vi "Get All DMA Data.vi"(10 "size":u32, 11 "arr":i32) -> (2 "function return":u32, 3 "arr out":i32)   [LabVIEW 2018, in "Copy of Andor SDK.lvlib"]
doc: "EXPNETTYPE unsigned int WINAPI GetAllDMAData(at_32 * arr, unsigned long size);"
uses:
  Copy of Andor SDK.lvlib
  <userlib>/Andor SDK/ATMCD32D.dll
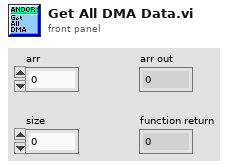
[diagram p1: front panel]
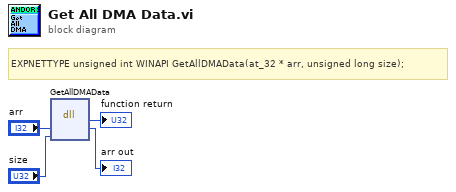
[diagram p0: block diagram]
diagram:
  # "EXPNETTYPE unsigned int WINAPI GetAllDMAData(at_32 * arr, unsigned long size);"
  n1 = dll-call lib="C:/Program Files (x86)/National Instruments/LabVIEW 2018/user.lib/Andor SDK/ATMCD32D.*" fn="GetAllDMAData"("arr"="arr", "size"="size") -> (→"function return":u32, "arr"=→"arr out":i32)  [unwired: 4 in, 2 out]
